vi "new_fail.vi"(8 "error out":errorcluster, 11 "reason":string) -> (3 "result":T1)   [LabVIEW 2015]
uses:
  tester_result.ctl
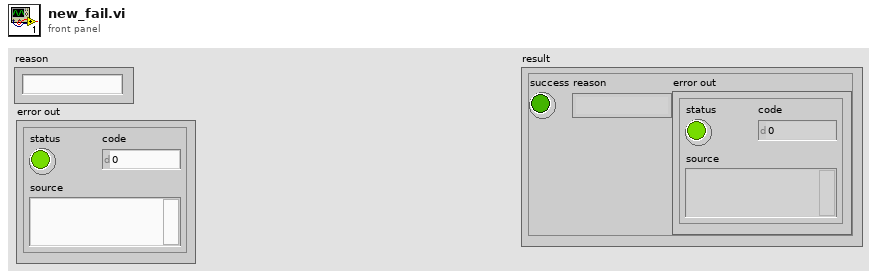
[diagram p1: front panel]
types:
  T1 = typedef "tester_result.ctl" = cluster{"success":bool, "reason":string, "error out":errorcluster}
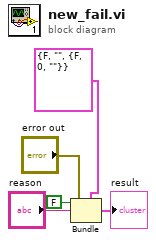
[diagram p0: block diagram]
diagram:
  n1 = Bundle(cluster=T1 {"success"=FALSE, "reason"="", "error out"={"status"=FALSE, "code"=0, "source"=""}} ("test_result"), "success"=FALSE, "reason"="reason", "error out"="error out") -> (→"result":T1)
